vi "To String.vi"(11 "AbstractDstarNode.lvclass in":refnum<class "NI_Robotics_AbstractDstarNode.lvclass">) -> (2 "output":T1, 3 "AbstractDstarNode.lvclass out":refnum<class "NI_Robotics_AbstractDstarNode.lvclass">)   [LabVIEW 2017, in "NI_Robotics_AbstractDstarNode.lvclass"]
uses:
  <vilib>/robotics/Navigation/shared/MapNode/AbstractDstarNode/NI_Robotics_AbstractDstarNode.lvclass
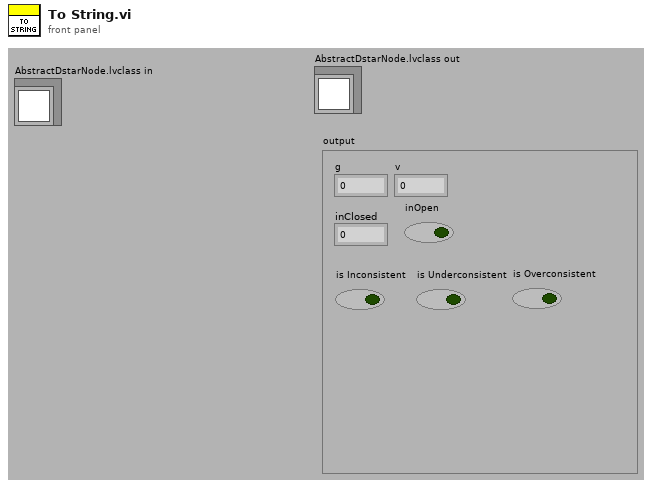
[diagram p1: front panel]
types:
  T1 = cluster{"g":dbl, "v":dbl, "inClosed":i32, "inOpen":bool, "is Inconsistent":bool, "is Underconsistent":bool, "is Overconsistent":bool}
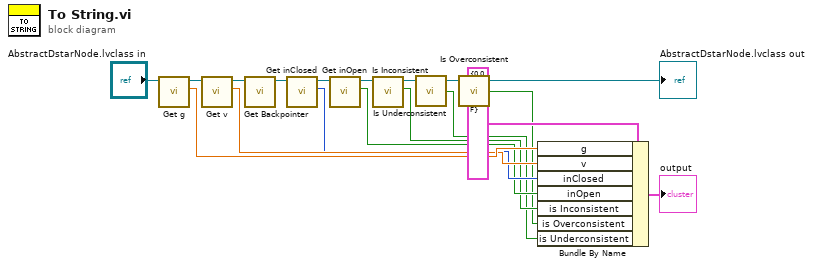
[diagram p0: block diagram]
diagram:
  n1 = call <vilib>:"Get g.vi"("AbstractDstarNode in"="AbstractDstarNode.lvclass in") -> ("g"=w8:dbl, "AbstractDstarNode out"=w17:refnum<class "NI_Robotics_AbstractDstarNode.lvclass">)  [unwired: 9 in]
  n2 = call <vilib>:"Get v.vi"("AbstractDstarNode in"=w17) -> ("v"=w7:dbl, "AbstractDstarNode out"=w16:refnum<class "NI_Robotics_AbstractDstarNode.lvclass">)  [unwired: 9 in]
  n3 = call <vilib>:"Get Backpointer.vi"("AbstractDstarNode in"=w16) -> ("AbstractDstarNode out"=w15:refnum<class "NI_Robotics_AbstractDstarNode.lvclass">)  [unwired: 8 in, 2 out]
  n4 = call <vilib>:"Get inClosed.vi"("AbstractDstarNode in"=w15) -> ("inClosed"=w6:i32, "AbstractDstarNode out"=w14:refnum<class "NI_Robotics_AbstractDstarNode.lvclass">)  [unwired: 8 in, 1 out]
  n5 = call <vilib>:"Get inOpen.vi"("AbstractDstarNode in"=w14) -> ("inOpen"=w5:bool, "AbstractDstarNode out"=w13:refnum<class "NI_Robotics_AbstractDstarNode.lvclass">)  [unwired: 8 in, 1 out]
  n6 = call <vilib>:"Is Inconsistent.vi"("AbstractDstarNode in"=w13) -> ("is Inconsistent"=w4:bool, "AbstractDstarNode out"=w12:refnum<class "NI_Robotics_AbstractDstarNode.lvclass">)  [unwired: 8 in, 1 out]
  n7 = call <vilib>:"Is Underconsistent.vi"("AbstractDstarNode in"=w12) -> ("is Underconsistent"=w2:bool, "AbstractDstarNode out"=w11:refnum<class "NI_Robotics_AbstractDstarNode.lvclass">)  [unwired: 2 in, 1 out]
  n8 = call <vilib>:"Is Overconsistent.vi"("AbstractDstarNode in"=w11) -> ("is Overconsistent"=w3:bool, "AbstractDstarNode out"=→"AbstractDstarNode.lvclass out":refnum<class "NI_Robotics_AbstractDstarNode.lvclass">)  [unwired: 2 in, 1 out]
  n9 = Bundle By Name(cluster=T1 {"g"=0.0, "v"=0.0, "inClosed"=0, "inOpen"=FALSE, "is Inconsistent"=FALSE, "is Underconsistent"=FALSE, "is Overconsistent"=FALSE} ("output 2"), "g"=w8, "v"=w7, "inClosed"=w6, "inOpen"=w5, "is Inconsistent"=w4, "is Overconsistent"=w3, "is Underconsistent"=w2) -> (→"output":T1)
